vi "Lab Panel V4.82.vi"() -> ()   [LabVIEW 2013] (continued)
                            n2114 = local write "ON L04-2"(w3494) -> ()
                          }
                        }
                      }
                      frame #1 {
                        n2115 = Unbundle(w3502) -> ("amps"=w3501:dbl, "volts"=w3500:dbl, "pf"=w3499:dbl)
                        n2116 = case shown="True" w3503 {
                          tunnel: w3510 -> [_ w3542]
                          tunnel: w3509 -> [_ w3549]
                          tunnel: w3508 -> [_ _]
                          tunnel: w3507 -> [_ _]
                          tunnel: w3506 -> [_ w3548]
                          tunnel: w3505 -> [_ w3547]
                          tunnel: w3504 -> [_ w3512]
                          tunnel: w3501 -> [_ w3544]
                          tunnel: w3500 -> [_ w3543]
                          tunnel: w3499 -> [_ w3541]
                          tunnel: w3498 -> [_ w3533]
                          frame False {
                          }
                          frame True {
                            n2117 = local read "TDMS LAB04-2"() -> (w3546:refnum<k34>)
                            n2118 = Build Array(w3543) -> (w3538:dbl[])
                            n2119 = Build Array(w3541) -> (w3537:dbl[])
                            n2120 = Build Array(w3548) -> (w3536:dbl[])
                            n2121 = Build Array(w3549) -> (w3535:dbl[])
                            n2122 = Build Array(w3544) -> (w3540:dbl[])
                            n2123 = Build Array(w3542) -> (w3539:dbl[])
                            n2124 = Build Array(w3547) -> (w3534:dbl[])
                            n2125 = Build Array("AMPS ON", "AMPS OFF", "VOLTS", "PF", "TEMP Live", "TEMP Neut", "CYCLE") -> (w3517:string[])
                            n2126 = Bundle By Name("Y"=w3540, "t0"=w3533) -> (w3532:waveform(dbl))  [unwired: 1 in]
                            n2127 = Bundle By Name("Y"=w3539, "t0"=w3533) -> (w3531:waveform(dbl))  [unwired: 1 in]
                            n2128 = Bundle By Name("Y"=w3538, "t0"=w3533) -> (w3530:waveform(dbl))  [unwired: 1 in]
                            n2129 = Bundle By Name("Y"=w3537, "t0"=w3533) -> (w3529:waveform(dbl))  [unwired: 1 in]
                            n2130 = Bundle By Name("Y"=w3536, "t0"=w3533) -> (w3528:waveform(dbl))  [unwired: 1 in]
                            n2131 = Bundle By Name("Y"=w3535, "t0"=w3533) -> (w3527:waveform(dbl))  [unwired: 1 in]
                            n2132 = Bundle By Name("Y"=w3534, "t0"=w3533) -> (w3526:waveform(dbl))  [unwired: 1 in]
                            n2133 = Build Array(w3532, w3531, w3530, w3529, w3528, w3527, w3526) -> (w3525:waveform(dbl)[])
                            n2134 = TDMS Write(0:w3546, 5:"TEST VALUES", 7:w3517, 9:w3525) -> (4:w3516:refnum<k34>, 6:w3515:string, 15:w3514:errorcluster)  [unwired: 2 in, 1 out]
                            n2135 = TDMS Write(0:w3516, 5:w3515, 7:"TIME", 9:w3512, 11:w3514) -> (15:w3511:errorcluster)  [unwired: 1 in, 3 out]
                            n2136 = local write "data file error"(w3511) -> ()
                          }
                        }
                      }
                    }
                  }
                }
              }
              frame #8 {
                n2137 = case shown="True" w3550 {
                  tunnel: w3554 -> [_ w3559]
                  tunnel: w3553 -> [_ w3558]
                  tunnel: w3552 -> [_ w3556]
                  tunnel: w3551 -> [_ w3555]
                  frame False {
                  }
                  frame True {
                    n2138 = local read "DISP LAB05-1"() -> (w3560:T4)
                    n2139 = local read "SIG LAB05-1"() -> (w3561:T2)
                    n2140 = local read "ON L05-1"() -> (w3557:cluster{"amps":dbl, "volts":dbl, "pf":dbl})
                    n2141 = Unbundle(w3561) -> ("AMPS"=w3567:dbl, "VOLTS"=w3565:dbl, "PF"=w3564:dbl, "Tmp Live"=w3563:dbl, "Tmp Neut"=w3566:dbl)
                    n2142 = Unbundle(w3560) -> ("CYCLE"=w3562:dbl)  [unwired: 2 out]
                    n2143 = stacked-sequence {
                      tunnel: w3567 -> [w3571 w3590]
                      tunnel: w3566 -> [_ w3589]
                      tunnel: w3565 -> [w3570 w3588]
                      tunnel: w3564 -> [w3569 w3587]
                      tunnel: w3563 -> [_ w3586]
                      tunnel: w3562 -> [_ w3585]
                      tunnel: w3559 -> [_ w3584]
                      tunnel: w3558 -> [w3572 _]
                      tunnel: w3557 -> [w3568 w3582]
                      tunnel: w3556 -> [_ w3583]
                      tunnel: w3555 -> [_ w3578]
                      frame #0 {
                        n2144 = case shown="True" w3572 {
                          tunnel: w3571 -> [_ w3577]
                          tunnel: w3570 -> [_ w3576]
                          tunnel: w3569 -> [_ w3575]
                          tunnel: w3568 -> [_ w3573]
                          frame False {
                          }
                          frame True {
                            n2145 = Bundle(cluster=w3573, "amps"=w3577, "volts"=w3576, "pf"=w3575) -> (w3574:cluster{"amps":dbl, "volts":dbl, "pf":dbl})
                            n2146 = local write "ON L05-1"(w3574) -> ()
                          }
                        }
                      }
                      frame #1 {
                        n2147 = Unbundle(w3582) -> ("amps"=w3581:dbl, "volts"=w3580:dbl, "pf"=w3579:dbl)
                        n2148 = case shown="True" w3583 {
                          tunnel: w3590 -> [_ w3622]
                          tunnel: w3589 -> [_ w3629]
                          tunnel: w3588 -> [_ _]
                          tunnel: w3587 -> [_ _]
                          tunnel: w3586 -> [_ w3628]
                          tunnel: w3585 -> [_ w3627]
                          tunnel: w3584 -> [_ w3592]
                          tunnel: w3581 -> [_ w3624]
                          tunnel: w3580 -> [_ w3623]
                          tunnel: w3579 -> [_ w3621]
                          tunnel: w3578 -> [_ w3613]
                          frame False {
                          }
                          frame True {
                            n2149 = local read "TDMS LAB05-1"() -> (w3626:refnum<k34>)
                            n2150 = Build Array(w3623) -> (w3618:dbl[])
                            n2151 = Build Array(w3621) -> (w3617:dbl[])
                            n2152 = Build Array(w3628) -> (w3616:dbl[])
                            n2153 = Build Array(w3629) -> (w3615:dbl[])
                            n2154 = Build Array(w3624) -> (w3620:dbl[])
                            n2155 = Build Array(w3622) -> (w3619:dbl[])
                            n2156 = Build Array(w3627) -> (w3614:dbl[])
                            n2157 = Build Array("AMPS ON", "AMPS OFF", "VOLTS", "PF", "TEMP Live", "TEMP Neut", "CYCLE") -> (w3597:string[])
                            n2158 = Bundle By Name("Y"=w3620, "t0"=w3613) -> (w3612:waveform(dbl))  [unwired: 1 in]
                            n2159 = Bundle By Name("Y"=w3619, "t0"=w3613) -> (w3611:waveform(dbl))  [unwired: 1 in]
                            n2160 = Bundle By Name("Y"=w3618, "t0"=w3613) -> (w3610:waveform(dbl))  [unwired: 1 in]
                            n2161 = Bundle By Name("Y"=w3617, "t0"=w3613) -> (w3609:waveform(dbl))  [unwired: 1 in]
                            n2162 = Bundle By Name("Y"=w3616, "t0"=w3613) -> (w3608:waveform(dbl))  [unwired: 1 in]
                            n2163 = Bundle By Name("Y"=w3615, "t0"=w3613) -> (w3607:waveform(dbl))  [unwired: 1 in]
                            n2164 = Bundle By Name("Y"=w3614, "t0"=w3613) -> (w3606:waveform(dbl))  [unwired: 1 in]
                            n2165 = Build Array(w3612, w3611, w3610, w3609, w3608, w3607, w3606) -> (w3605:waveform(dbl)[])
                            n2166 = TDMS Write(0:w3626, 5:"TEST VALUES", 7:w3597, 9:w3605) -> (4:w3596:refnum<k34>, 6:w3595:string, 15:w3594:errorcluster)  [unwired: 2 in, 1 out]
                            n2167 = TDMS Write(0:w3596, 5:w3595, 7:"TIME", 9:w3592, 11:w3594) -> (15:w3591:errorcluster)  [unwired: 1 in, 3 out]
                            n2168 = local write "data file error"(w3591) -> ()
                          }
                        }
                      }
                    }
                  }
                }
              }
              frame #9 {
                n2169 = case shown="True" w3630 {
                  tunnel: w3634 -> [_ w3639]
                  tunnel: w3633 -> [_ w3638]
                  tunnel: w3632 -> [_ w3636]
                  tunnel: w3631 -> [_ w3635]
                  frame False {
                  }
                  frame True {
                    n2170 = local read "DISP LAB05-2"() -> (w3640:T4)
                    n2171 = local read "SIG LAB05-2"() -> (w3641:T2)
                    n2172 = local read "ON L05-2"() -> (w3637:cluster{"amps":dbl, "volts":dbl, "pf":dbl})
                    n2173 = Unbundle(w3641) -> ("AMPS"=w3647:dbl, "VOLTS"=w3645:dbl, "PF"=w3644:dbl, "Tmp Live"=w3643:dbl, "Tmp Neut"=w3646:dbl)
                    n2174 = Unbundle(w3640) -> ("CYCLE"=w3642:dbl)  [unwired: 2 out]
                    n2175 = stacked-sequence {
                      tunnel: w3647 -> [w3651 w3670]
                      tunnel: w3646 -> [_ w3669]
                      tunnel: w3645 -> [w3650 w3668]
                      tunnel: w3644 -> [w3649 w3667]
                      tunnel: w3643 -> [_ w3666]
                      tunnel: w3642 -> [_ w3665]
                      tunnel: w3639 -> [_ w3664]
                      tunnel: w3638 -> [w3652 _]
                      tunnel: w3637 -> [w3648 w3662]
                      tunnel: w3636 -> [_ w3663]
                      tunnel: w3635 -> [_ w3658]
                      frame #0 {
                        n2176 = case shown="True" w3652 {
                          tunnel: w3651 -> [_ w3657]
                          tunnel: w3650 -> [_ w3656]
                          tunnel: w3649 -> [_ w3655]
                          tunnel: w3648 -> [_ w3653]
                          frame False {
                          }
                          frame True {
                            n2177 = Bundle(cluster=w3653, "amps"=w3657, "volts"=w3656, "pf"=w3655) -> (w3654:cluster{"amps":dbl, "volts":dbl, "pf":dbl})
                            n2178 = local write "ON L05-2"(w3654) -> ()
                          }
                        }
                      }
                      frame #1 {
                        n2179 = Unbundle(w3662) -> ("amps"=w3661:dbl, "volts"=w3660:dbl, "pf"=w3659:dbl)
                        n2180 = case shown="True" w3663 {
                          tunnel: w3670 -> [_ w3702]
                          tunnel: w3669 -> [_ w3709]
                          tunnel: w3668 -> [_ _]
                          tunnel: w3667 -> [_ _]
                          tunnel: w3666 -> [_ w3708]
                          tunnel: w3665 -> [_ w3707]
                          tunnel: w3664 -> [_ w3672]
                          tunnel: w3661 -> [_ w3704]
                          tunnel: w3660 -> [_ w3703]
                          tunnel: w3659 -> [_ w3701]
                          tunnel: w3658 -> [_ w3693]
                          frame False {
                          }
                          frame True {
                            n2181 = local read "TDMS LAB05-2"() -> (w3706:refnum<k34>)
                            n2182 = Build Array(w3703) -> (w3698:dbl[])
                            n2183 = Build Array(w3701) -> (w3697:dbl[])
                            n2184 = Build Array(w3708) -> (w3696:dbl[])
                            n2185 = Build Array(w3709) -> (w3695:dbl[])
                            n2186 = Build Array(w3704) -> (w3700:dbl[])
                            n2187 = Build Array(w3702) -> (w3699:dbl[])
                            n2188 = Build Array(w3707) -> (w3694:dbl[])
                            n2189 = Build Array("AMPS ON", "AMPS OFF", "VOLTS", "PF", "TEMP Live", "TEMP Neut", "CYCLE") -> (w3677:string[])
                            n2190 = Bundle By Name("Y"=w3700, "t0"=w3693) -> (w3692:waveform(dbl))  [unwired: 1 in]
                            n2191 = Bundle By Name("Y"=w3699, "t0"=w3693) -> (w3691:waveform(dbl))  [unwired: 1 in]
                            n2192 = Bundle By Name("Y"=w3698, "t0"=w3693) -> (w3690:waveform(dbl))  [unwired: 1 in]
                            n2193 = Bundle By Name("Y"=w3697, "t0"=w3693) -> (w3689:waveform(dbl))  [unwired: 1 in]
                            n2194 = Bundle By Name("Y"=w3696, "t0"=w3693) -> (w3688:waveform(dbl))  [unwired: 1 in]
                            n2195 = Bundle By Name("Y"=w3695, "t0"=w3693) -> (w3687:waveform(dbl))  [unwired: 1 in]
                            n2196 = Bundle By Name("Y"=w3694, "t0"=w3693) -> (w3686:waveform(dbl))  [unwired: 1 in]
                            n2197 = Build Array(w3692, w3691, w3690, w3689, w3688, w3687, w3686) -> (w3685:waveform(dbl)[])
                            n2198 = TDMS Write(0:w3706, 5:"TEST VALUES", 7:w3677, 9:w3685) -> (4:w3676:refnum<k34>, 6:w3675:string, 15:w3674:errorcluster)  [unwired: 2 in, 1 out]
                            n2199 = TDMS Write(0:w3676, 5:w3675, 7:"TIME", 9:w3672, 11:w3674) -> (15:w3671:errorcluster)  [unwired: 1 in, 3 out]
                            n2200 = local write "data file error"(w3671) -> ()
                          }
                        }
                      }
                    }
                  }
                }
              }
            }
          }
          frame #13 {
            # "display test values on chart"
            n2201 = case shown="\"OFF CYCLE\"" "Select  Cycle" {
              tunnel: [1 w3715] -> w3710
              frame "ON CYCLE", Default {
              }
              frame "OFF CYCLE" {
                n2202 = local read "on loops"() -> (w3717:dbl)
                n2203 = Add(x=w3717, y=2) -> (x+y=w3715:dbl)
              }
            }
            n2204 = local read "jig cycle"() -> (w3712:dbl)
            n2205 = Equal?(x=w3712, y=w3710) -> (x = y?=w3713:bool)
            n2206 = case shown="True" w3713 {
              frame False {
              }
              frame True {
                n2207 = local read "SIG LAB05-1"() -> (w3759:T2)
                n2208 = local read "SIG LAB04-2"() -> (w3760:T2)
                n2209 = local read "SIG LAB05-2"() -> (w3758:T2)
                n2210 = local read "SIG LAB04-1"() -> (w3761:T2)
                n2211 = local read "SIG LAB03-1"() -> (w3763:T2)
                n2212 = local read "SIG LAB03-2"() -> (w3762:T2)
                n2213 = local read "SIG LAB01-1"() -> (w3767:T2)
                n2214 = local read "SIG LAB02-2"() -> (w3764:T2)
                n2215 = local read "SIG LAB02-1"() -> (w3765:T2)
                n2216 = local read "SIG LAB01-2"() -> (w3766:T2)
                n2217 = Unbundle(w3760) -> ("AMPS"=w3750:dbl, "VOLTS"=w3740:dbl, "Tmp Live"=w3730:dbl, "Tmp Neut"=w3720:dbl)  [unwired: 1 out]
                n2218 = Unbundle(w3759) -> ("AMPS"=w3749:dbl, "VOLTS"=w3739:dbl, "Tmp Live"=w3729:dbl, "Tmp Neut"=w3719:dbl)  [unwired: 1 out]
                n2219 = Unbundle(w3758) -> ("AMPS"=w3748:dbl, "VOLTS"=w3738:dbl, "Tmp Live"=w3728:dbl, "Tmp Neut"=w3718:dbl)  [unwired: 1 out]
                n2220 = Unbundle(w3761) -> ("AMPS"=w3751:dbl, "VOLTS"=w3741:dbl, "Tmp Live"=w3731:dbl, "Tmp Neut"=w3721:dbl)  [unwired: 1 out]
                n2221 = Unbundle(w3762) -> ("AMPS"=w3752:dbl, "VOLTS"=w3742:dbl, "Tmp Live"=w3732:dbl, "Tmp Neut"=w3722:dbl)  [unwired: 1 out]
                n2222 = Unbundle(w3763) -> ("AMPS"=w3753:dbl, "VOLTS"=w3743:dbl, "Tmp Live"=w3733:dbl, "Tmp Neut"=w3723:dbl)  [unwired: 1 out]
                n2223 = Unbundle(w3764) -> ("AMPS"=w3754:dbl, "VOLTS"=w3744:dbl, "Tmp Live"=w3734:dbl, "Tmp Neut"=w3724:dbl)  [unwired: 1 out]
                n2224 = Unbundle(w3765) -> ("AMPS"=w3755:dbl, "VOLTS"=w3745:dbl, "Tmp Live"=w3735:dbl, "Tmp Neut"=w3725:dbl)  [unwired: 1 out]
                n2225 = Unbundle(w3767) -> ("AMPS"=w3757:dbl, "VOLTS"=w3747:dbl, "Tmp Live"=w3737:dbl, "Tmp Neut"=w3727:dbl)  [unwired: 1 out]
                n2226 = Unbundle(w3766) -> ("AMPS"=w3756:dbl, "VOLTS"=w3746:dbl, "Tmp Live"=w3736:dbl, "Tmp Neut"=w3726:dbl)  [unwired: 1 out]
                n2227 = stacked-sequence {
                  tunnel: w3757 -> [w3778 _ _ _]
                  tunnel: w3756 -> [w3777 _ _ _]
                  tunnel: w3755 -> [w3776 _ _ _]
                  tunnel: w3754 -> [w3775 _ _ _]
                  tunnel: w3753 -> [w3774 _ _ _]
                  tunnel: w3752 -> [w3773 _ _ _]
                  tunnel: w3751 -> [w3772 _ _ _]
                  tunnel: w3750 -> [w3771 _ _ _]
                  tunnel: w3749 -> [w3770 _ _ _]
                  tunnel: w3748 -> [w3769 _ _ _]
                  tunnel: w3747 -> [_ w3789 _ _]
                  tunnel: w3746 -> [_ w3788 _ _]
                  tunnel: w3745 -> [_ w3787 _ _]
                  tunnel: w3744 -> [_ w3786 _ _]
                  tunnel: w3743 -> [_ w3785 _ _]
                  tunnel: w3742 -> [_ w3784 _ _]
                  tunnel: w3741 -> [_ w3783 _ _]
                  tunnel: w3740 -> [_ w3782 _ _]
                  tunnel: w3739 -> [_ w3781 _ _]
                  tunnel: w3738 -> [_ w3780 _ _]
                  tunnel: w3737 -> [_ _ w3800 _]
                  tunnel: w3736 -> [_ _ w3799 _]
                  tunnel: w3735 -> [_ _ w3798 _]
                  tunnel: w3734 -> [_ _ w3797 _]
                  tunnel: w3733 -> [_ _ w3796 _]
                  tunnel: w3732 -> [_ _ w3795 _]
                  tunnel: w3731 -> [_ _ w3794 _]
                  tunnel: w3730 -> [_ _ w3793 _]
                  tunnel: w3729 -> [_ _ w3792 _]
                  tunnel: w3728 -> [_ _ w3791 _]
                  tunnel: w3727 -> [_ _ _ w3811]
                  tunnel: w3726 -> [_ _ _ w3810]
                  tunnel: w3725 -> [_ _ _ w3809]
                  tunnel: w3724 -> [_ _ _ w3808]
                  tunnel: w3723 -> [_ _ _ w3807]
                  tunnel: w3722 -> [_ _ _ w3806]
                  tunnel: w3721 -> [_ _ _ w3805]
                  tunnel: w3720 -> [_ _ _ w3804]
                  tunnel: w3719 -> [_ _ _ w3803]
                  tunnel: w3718 -> [_ _ _ w3802]
                  frame #0 {
                    n2228 = Bundle("AMPS"=w3778, "AMPS"=w3777, "AMPS"=w3776, "AMPS"=w3775, "AMPS"=w3774, "AMPS"=w3773, "AMPS"=w3772, "AMPS"=w3771, "AMPS"=w3770, "AMPS"=w3769) -> (→"TEST AMPS CHART":T6)  [unwired: 1 in]
                  }
                  frame #1 {
                    n2229 = Bundle("VOLTS"=w3789, "VOLTS"=w3788, "VOLTS"=w3787, "VOLTS"=w3786, "VOLTS"=w3785, "VOLTS"=w3784, "VOLTS"=w3783, "VOLTS"=w3782, "VOLTS"=w3781, "VOLTS"=w3780) -> (→"TEST VOLTS CHART":T29)  [unwired: 1 in]
                  }
                  frame #2 {
                    n2230 = Bundle("Tmp Live"=w3800, "Tmp Live"=w3799, "Tmp Live"=w3798, "Tmp Live"=w3797, "Tmp Live"=w3796, "Tmp Live"=w3795, "Tmp Live"=w3794, "Tmp Live"=w3793, "Tmp Live"=w3792, "Tmp Live"=w3791) -> (→"TEMPERATURE (L) CHART":T30)  [unwired: 1 in]
                  }
                  frame #3 {
                    n2231 = Bundle("Tmp Neut"=w3811, "Tmp Neut"=w3810, "Tmp Neut"=w3809, "Tmp Neut"=w3808, "Tmp Neut"=w3807, "Tmp Neut"=w3806, "Tmp Neut"=w3805, "Tmp Neut"=w3804, "Tmp Neut"=w3803, "Tmp Neut"=w3802) -> (→"TEMPERATURE (N) CHART":T31)  [unwired: 1 in]
                  }
                }
              }
            }
          }
          frame #14 {
            # "check for amps fail"
            # "check for cycle test & temperature rise fail conditions"
            n2232 = local read "on loops"() -> (w3838:dbl)
            n2233 = local read "jig cycle"() -> (w3835:dbl)
            n2234 = local read "jig cycle"() -> (w3840:dbl)
            n2235 = Add(x=w3838, y=3.0) -> (x+y=w3836:dbl)
            n2236 = Equal?(x=w3835, y=w3836) -> (x = y?=w3831:bool)
            n2237 = local read "Fail Loops"() -> (w3812:dbl)
            n2238 = Equal?(x=w3840, y=1.0) -> (x = y?=w3833:bool)
            n2239 = global write "Global 1.vi" "fail count"(w3812) -> ()
            n2240 = stacked-sequence {
              tunnel: w3834 -> [w3843 _ _ _ _ _ _ _ _ _]
              tunnel: w3833 -> [w3844 w3864 w3884 w3904 w3924 w3944 w3964 w3984 w4004 w4024]
              tunnel: w3832 -> [w3841 _ _ _ _ _ _ _ _ _]
              tunnel: w3831 -> [w3842 w3863 w3883 w3903 w3923 w3943 w3963 w3983 w4003 w4023]
              tunnel: w3830 -> [_ w3862 _ _ _ _ _ _ _ _]
              tunnel: w3829 -> [_ w3861 _ _ _ _ _ _ _ _]
              tunnel: w3828 -> [_ _ w3882 _ _ _ _ _ _ _]
              tunnel: w3827 -> [_ _ w3881 _ _ _ _ _ _ _]
              tunnel: w3826 -> [_ _ _ w3902 _ _ _ _ _ _]
              tunnel: w3825 -> [_ _ _ w3901 _ _ _ _ _ _]
              tunnel: w3824 -> [_ _ _ _ w3922 _ _ _ _ _]
              tunnel: w3823 -> [_ _ _ _ w3921 _ _ _ _ _]
              tunnel: w3822 -> [_ _ _ _ _ w3942 _ _ _ _]
              tunnel: w3821 -> [_ _ _ _ _ w3941 _ _ _ _]
              tunnel: w3820 -> [_ _ _ _ _ _ w3962 _ _ _]
              tunnel: w3819 -> [_ _ _ _ _ _ w3961 _ _ _]
              tunnel: w3818 -> [_ _ _ _ _ _ _ w3982 _ _]
              tunnel: w3817 -> [_ _ _ _ _ _ _ w3981 _ _]
              tunnel: w3816 -> [_ _ _ _ _ _ _ _ w4002 _]
              tunnel: w3815 -> [_ _ _ _ _ _ _ _ w4001 _]
              tunnel: w3814 -> [_ _ _ _ _ _ _ _ _ w4022]
              tunnel: w3813 -> [_ _ _ _ _ _ _ _ _ w4021]
              frame #0 {
                # "LAB01-1"
                n2241 = case shown="True" w3841 {
                  tunnel: w3844 -> [_ w3857]
                  tunnel: w3843 -> [_ w3854]
                  tunnel: w3842 -> [_ w3853]
                  frame False {
                  }
                  frame True {
                    n2242 = local read "TEMP START LAB01-1"() -> (w3859:cluster{"TL":dbl, "TN":dbl})
                    n2243 = local read "RESULT LAB01-1"() -> (w3848:bool)
                    n2244 = local read "FAIL LAB01-1"() -> (w3851:cluster{"LO":dbl, "HI":dbl})
                    n2245 = local read "TDMS LAB01-1"() -> (w3858:refnum<k34>)
                    n2246 = local read "SET LAB01-1"() -> (w3855:T5)
                    n2247 = local read "DISP LAB01-1"() -> (w3856:T4)
                    n2248 = local read "SIG LAB01-1"() -> (w3860:T2)
                    n2249 = Bundle("FAIL LAB01-1"=w3851, "SIG LAB01-1"=w3860, "TEMP START LAB01-1"=w3859, "DISP LAB01-1"=w3856, "SET LAB01-1"=w3855, "TDMS LAB01-1"=w3858) -> (w3845:T32)  [unwired: 1 in]
                    n2250 = call "sub vi - cycle&temp fail v6.vi"("Amps Lo?"=w3857, "Input Cluster"=w3845, "SELECT"=w3854, "Amps Hi?"=w3853, "Result In"=w3848) -> ("(FAIL) out"=w3850:cluster{"FAIL LO":dbl, "FAIL HI":dbl}, "(DISP) out"=w3846:T4, "T-RISE"=w3847:cluster{"T-RISE (L)":dbl, "T-RISE (N)":dbl}, "Result Out"=w3849:bool, "file error"=w3852:errorcluster)  [unwired: 10 in]
                    n2251 = local write "TEMP RISE LAB01-1"(w3847) -> ()
                    n2252 = local write "FAIL LAB01-1"(w3850) -> ()
                    n2253 = local write "DISP LAB01-1"(w3846) -> ()
                    n2254 = local write "RESULT LAB01-1"(w3849) -> ()
                    n2255 = local write "data file error"(w3852) -> ()
                  }
                }
              }
              frame #1 {
                # "LAB01-2"
                n2256 = case shown="True" w3862 {
                  tunnel: w3864 -> [_ w3877]
                  tunnel: w3861 -> [_ w3874]
                  tunnel: w3863 -> [_ w3873]
                  frame False {
                  }
                  frame True {
                    n2257 = local read "TEMP START LAB01-2"() -> (w3879:cluster{"TL":dbl, "TN":dbl})
                    n2258 = local read "FAIL LAB01-2"() -> (w3870:cluster{"LO":dbl, "HI":dbl})
                    n2259 = local read "TDMS LAB01-2"() -> (w3878:refnum<k34>)
                    n2260 = local read "SET LAB01-2"() -> (w3875:T5)
                    n2261 = local read "DISP LAB01-2"() -> (w3876:T4)
                    n2262 = local read "RESULT LAB01-2"() -> (w3867:bool)
                    n2263 = local read "SIG LAB01-2"() -> (w3880:T2)
                    n2264 = Bundle("FAIL LAB01-2"=w3870, "SIG LAB01-2"=w3880, "TEMP START LAB01-2"=w3879, "DISP LAB01-2"=w3876, "SET LAB01-2"=w3875, "TDMS LAB01-2"=w3878) -> (w3865:T33)  [unwired: 1 in]
                    n2265 = call "sub vi - cycle&temp fail v6.vi"("Amps Lo?"=w3877, "Input Cluster"=w3865, "SELECT"=w3874, "Amps Hi?"=w3873, "Result In"=w3867) -> ("(FAIL) out"=w3869:cluster{"FAIL LO":dbl, "FAIL HI":dbl}, "(DISP) out"=w3872:T4, "T-RISE"=w3866:cluster{"T-RISE (L)":dbl, "T-RISE (N)":dbl}, "Result Out"=w3868:bool, "file error"=w3871:errorcluster)  [unwired: 10 in]
                    n2266 = local write "TEMP RISE LAB01-2"(w3866) -> ()
                    n2267 = local write "FAIL LAB01-2"(w3869) -> ()
                    n2268 = local write "DISP LAB01-2"(w3872) -> ()
                    n2269 = local write "RESULT LAB01-2"(w3868) -> ()
                    n2270 = local write "data file error"(w3871) -> ()
                  }
                }
              }
              frame #2 {
                # "LAB02-1"
                n2271 = case shown="True" w3882 {
                  tunnel: w3884 -> [_ w3897]
                  tunnel: w3881 -> [_ w3894]
                  tunnel: w3883 -> [_ w3893]
                  frame False {
                  }
                  frame True {
                    n2272 = local read "TEMP START LAB02-1"() -> (w3899:cluster{"TL":dbl, "TN":dbl})
                    n2273 = local read "FAIL LAB02-1"() -> (w3890:cluster{"LO":dbl, "HI":dbl})
                    n2274 = local read "TDMS LAB02-1"() -> (w3898:refnum<k34>)
                    n2275 = local read "SET LAB02-1"() -> (w3895:T5)
                    n2276 = local read "DISP LAB02-1"() -> (w3896:T4)
                    n2277 = local read "SIG LAB02-1"() -> (w3900:T2)
                    n2278 = local read "RESULT LAB02-1"() -> (w3887:bool)
                    n2279 = Bundle("FAIL LAB02-1"=w3890, "SIG LAB02-1"=w3900, "TEMP START LAB02-1"=w3899, "DISP LAB02-1"=w3896, "SET LAB02-1"=w3895, "TDMS LAB02-1"=w3898) -> (w3885:T34)  [unwired: 1 in]
                    n2280 = call "sub vi - cycle&temp fail v6.vi"("Amps Lo?"=w3897, "Input Cluster"=w3885, "SELECT"=w3894, "Amps Hi?"=w3893, "Result In"=w3887) -> ("(FAIL) out"=w3889:cluster{"FAIL LO":dbl, "FAIL HI":dbl}, "(DISP) out"=w3892:T4, "T-RISE"=w3886:cluster{"T-RISE (L)":dbl, "T-RISE (N)":dbl}, "Result Out"=w3888:bool, "file error"=w3891:errorcluster)  [unwired: 10 in]
                    n2281 = local write "TEMP RISE LAB02-1"(w3886) -> ()
                    n2282 = local write "FAIL LAB02-1"(w3889) -> ()
                    n2283 = local write "DISP LAB02-1"(w3892) -> ()
                    n2284 = local write "RESULT LAB02-1"(w3888) -> ()
                    n2285 = local write "data file error"(w3891) -> ()
                  }
                }
              }
              frame #3 {
                # "LAB02-2"
                n2286 = case shown="True" w3902 {
                  tunnel: w3904 -> [_ w3917]
                  tunnel: w3901 -> [_ w3914]
                  tunnel: w3903 -> [_ w3913]
                  frame False {
                  }
                  frame True {
                    n2287 = local read "TEMP START LAB02-2"() -> (w3919:cluster{"TL":dbl, "TN":dbl})
                    n2288 = local read "FAIL LAB02-2"() -> (w3910:cluster{"LO":dbl, "HI":dbl})
                    n2289 = local read "TDMS LAB02-2"() -> (w3918:refnum<k34>)
                    n2290 = local read "SET LAB02-2"() -> (w3915:T5)
                    n2291 = local read "DISP LAB02-2"() -> (w3916:T4)
                    n2292 = local read "SIG LAB02-2"() -> (w3920:T2)
                    n2293 = local read "RESULT LAB02-2"() -> (w3907:bool)
                    n2294 = Bundle("FAIL LAB02-2"=w3910, "SIG LAB02-2"=w3920, "TEMP START LAB02-2"=w3919, "DISP LAB02-2"=w3916, "SET LAB02-2"=w3915, "TDMS LAB02-2"=w3918) -> (w3905:T35)  [unwired: 1 in]
                    n2295 = call "sub vi - cycle&temp fail v6.vi"("Amps Lo?"=w3917, "Input Cluster"=w3905, "SELECT"=w3914, "Amps Hi?"=w3913, "Result In"=w3907) -> ("(FAIL) out"=w3909:cluster{"FAIL LO":dbl, "FAIL HI":dbl}, "(DISP) out"=w3912:T4, "T-RISE"=w3906:cluster{"T-RISE (L)":dbl, "T-RISE (N)":dbl}, "Result Out"=w3908:bool, "file error"=w3911:errorcluster)  [unwired: 10 in]
                    n2296 = local write "TEMP RISE LAB02-2"(w3906) -> ()
                    n2297 = local write "FAIL LAB02-2"(w3909) -> ()
                    n2298 = local write "DISP LAB02-2"(w3912) -> ()
                    n2299 = local write "RESULT LAB02-2"(w3908) -> ()
                    n2300 = local write "data file error"(w3911) -> ()
                  }
                }
              }
              frame #4 {
                # "LAB03-1"
                n2301 = case shown="True" w3922 {
                  tunnel: w3924 -> [_ w3937]
                  tunnel: w3921 -> [_ w3934]
                  tunnel: w3923 -> [_ w3933]
                  frame False {
                  }
                  frame True {
                    n2302 = local read "TEMP START LAB03-1"() -> (w3939:cluster{"TL":dbl, "TN":dbl})
                    n2303 = local read "FAIL LAB03-1"() -> (w3930:cluster{"LO":dbl, "HI":dbl})
                    n2304 = local read "TDMS LAB03-1"() -> (w3938:refnum<k34>)
                    n2305 = local read "SET LAB03-1"() -> (w3935:T5)
                    n2306 = local read "DISP LAB03-1"() -> (w3936:T4)
                    n2307 = local read "SIG LAB03-1"() -> (w3940:T2)
                    n2308 = local read "RESULT LAB03-1"() -> (w3927:bool)
                    n2309 = Bundle("FAIL LAB03-1"=w3930, "SIG LAB03-1"=w3940, "TEMP START LAB03-1"=w3939, "DISP LAB03-1"=w3936, "SET LAB03-1"=w3935, "TDMS LAB03-1"=w3938) -> (w3925:T36)  [unwired: 1 in]
                    n2310 = call "sub vi - cycle&temp fail v6.vi"("Amps Lo?"=w3937, "Input Cluster"=w3925, "SELECT"=w3934, "Amps Hi?"=w3933, "Result In"=w3927) -> ("(FAIL) out"=w3929:cluster{"FAIL LO":dbl, "FAIL HI":dbl}, "(DISP) out"=w3932:T4, "T-RISE"=w3926:cluster{"T-RISE (L)":dbl, "T-RISE (N)":dbl}, "Result Out"=w3928:bool, "file error"=w3931:errorcluster)  [unwired: 10 in]
                    n2311 = local write "TEMP RISE LAB03-1"(w3926) -> ()
                    n2312 = local write "FAIL LAB03-1"(w3929) -> ()
                    n2313 = local write "DISP LAB03-1"(w3932) -> ()
                    n2314 = local write "RESULT LAB03-1"(w3928) -> ()
                    n2315 = local write "data file error"(w3931) -> ()
                  }
                }
              }
              frame #5 {
                # "LAB03-2"
                n2316 = case shown="True" w3942 {
                  tunnel: w3944 -> [_ w3957]
                  tunnel: w3941 -> [_ w3954]
                  tunnel: w3943 -> [_ w3953]
                  frame False {
                  }
                  frame True {
                    n2317 = local read "TEMP START LAB03-2"() -> (w3959:cluster{"TL":dbl, "TN":dbl})
                    n2318 = local read "FAIL LAB03-2"() -> (w3950:cluster{"LO":dbl, "HI":dbl})
                    n2319 = local read "TDMS LAB03-2"() -> (w3958:refnum<k34>)
                    n2320 = local read "SET LAB03-2"() -> (w3955:T5)
                    n2321 = local read "DISP LAB03-2"() -> (w3956:T4)
                    n2322 = local read "RESULT LAB03-2"() -> (w3947:bool)
                    n2323 = local read "SIG LAB03-2"() -> (w3960:T2)
                    n2324 = Bundle("FAIL LAB03-2"=w3950, "SIG LAB03-2"=w3960, "TEMP START LAB03-2"=w3959, "DISP LAB03-2"=w3956, "SET LAB03-2"=w3955, "TDMS LAB03-2"=w3958) -> (w3945:T37)  [unwired: 1 in]
                    n2325 = call "sub vi - cycle&temp fail v6.vi"("Amps Lo?"=w3957, "Input Cluster"=w3945, "SELECT"=w3954, "Amps Hi?"=w3953, "Result In"=w3947) -> ("(FAIL) out"=w3949:cluster{"FAIL LO":dbl, "FAIL HI":dbl}, "(DISP) out"=w3952:T4, "T-RISE"=w3946:cluster{"T-RISE (L)":dbl, "T-RISE (N)":dbl}, "Result Out"=w3948:bool, "file error"=w3951:errorcluster)  [unwired: 10 in]
                    n2326 = local write "FAIL LAB03-2"(w3949) -> ()
                    n2327 = local write "TEMP RISE LAB03-2"(w3946) -> ()
                    n2328 = local write "DISP LAB03-2"(w3952) -> ()
                    n2329 = local write "RESULT LAB03-2"(w3948) -> ()
                    n2330 = local write "data file error"(w3951) -> ()
                  }
                }
              }
              frame #6 {
                # "LAB04-1"
                n2331 = case shown="True" w3962 {
                  tunnel: w3964 -> [_ w3977]
                  tunnel: w3961 -> [_ w3974]
                  tunnel: w3963 -> [_ w3973]
                  frame False {
                  }
                  frame True {
                    n2332 = local read "TEMP START LAB04-1"() -> (w3979:cluster{"TL":dbl, "TN":dbl})
                    n2333 = local read "FAIL LAB04-1"() -> (w3970:cluster{"LO":dbl, "HI":dbl})
                    n2334 = local read "TDMS LAB04-1"() -> (w3978:refnum<k34>)
                    n2335 = local read "SET LAB04-1"() -> (w3975:T5)
                    n2336 = local read "DISP LAB04-1"() -> (w3976:T4)
                    n2337 = local read "SIG LAB04-1"() -> (w3980:T2)
                    n2338 = local read "RESULT LAB04-1"() -> (w3967:bool)
                    n2339 = Bundle("FAIL LAB04-1"=w3970, "SIG LAB04-1"=w3980, "TEMP START LAB04-1"=w3979, "DISP LAB04-1"=w3976, "SET LAB04-1"=w3975, "TDMS LAB04-1"=w3978) -> (w3965:T38)  [unwired: 1 in]
                    n2340 = call "sub vi - cycle&temp fail v6.vi"("Amps Lo?"=w3977, "Input Cluster"=w3965, "SELECT"=w3974, "Amps Hi?"=w3973, "Result In"=w3967) -> ("(FAIL) out"=w3969:cluster{"FAIL LO":dbl, "FAIL HI":dbl}, "(DISP) out"=w3972:T4, "T-RISE"=w3966:cluster{"T-RISE (L)":dbl, "T-RISE (N)":dbl}, "Result Out"=w3968:bool, "file error"=w3971:errorcluster)  [unwired: 10 in]
                    n2341 = local write "TEMP RISE LAB04-1"(w3966) -> ()
                    n2342 = local write "FAIL LAB04-1"(w3969) -> ()
                    n2343 = local write "DISP LAB04-1"(w3972) -> ()
                    n2344 = local write "RESULT LAB04-1"(w3968) -> ()
                    n2345 = local write "data file error"(w3971) -> ()
                  }
                }
              }
              frame #7 {
                # "LAB04-2"
                n2346 = case shown="True" w3982 {
                  tunnel: w3984 -> [_ w3997]
                  tunnel: w3981 -> [_ w3994]
                  tunnel: w3983 -> [_ w3993]
                  frame False {
                  }
                  frame True {
                    n2347 = local read "TEMP START LAB04-2"() -> (w3999:cluster{"TL":dbl, "TN":dbl})
                    n2348 = local read "FAIL LAB04-2"() -> (w3990:cluster{"LO":dbl, "HI":dbl})
                    n2349 = local read "TDMS LAB04-2"() -> (w3998:refnum<k34>)
                    n2350 = local read "SET LAB04-2"() -> (w3995:T5)
                    n2351 = local read "DISP LAB04-2"() -> (w3996:T4)
                    n2352 = local read "SIG LAB04-2"() -> (w4000:T2)
                    n2353 = local read "RESULT LAB04-2"() -> (w3987:bool)
                    n2354 = Bundle("FAIL LAB04-2"=w3990, "SIG LAB04-2"=w4000, "TEMP START LAB04-2"=w3999, "DISP LAB04-2"=w3996, "SET LAB04-2"=w3995, "TDMS LAB04-2"=w3998) -> (w3985:T39)  [unwired: 1 in]
                    n2355 = call "sub vi - cycle&temp fail v6.vi"("Amps Lo?"=w3997, "Input Cluster"=w3985, "SELECT"=w3994, "Amps Hi?"=w3993, "Result In"=w3987) -> ("(FAIL) out"=w3989:cluster{"FAIL LO":dbl, "FAIL HI":dbl}, "(DISP) out"=w3992:T4, "T-RISE"=w3986:cluster{"T-RISE (L)":dbl, "T-RISE (N)":dbl}, "Result Out"=w3988:bool, "file error"=w3991:errorcluster)  [unwired: 10 in]
                    n2356 = local write "TEMP RISE LAB04-2"(w3986) -> ()
                    n2357 = local write "FAIL LAB04-2"(w3989) -> ()
                    n2358 = local write "DISP LAB04-2"(w3992) -> ()
                    n2359 = local write "RESULT LAB04-2"(w3988) -> ()
                    n2360 = local write "data file error"(w3991) -> ()
                  }
                }
              }
              frame #8 {
                # "LAB05-1"
                n2361 = case shown="True" w4002 {
                  tunnel: w4004 -> [_ w4017]
                  tunnel: w4001 -> [_ w4014]
                  tunnel: w4003 -> [_ w4013]
                  frame False {
                  }
                  frame True {
                    n2362 = local read "TEMP START LAB05-1"() -> (w4019:cluster{"TL":dbl, "TN":dbl})
                    n2363 = local read "FAIL LAB05-1"() -> (w4010:cluster{"LO":dbl, "HI":dbl})
                    n2364 = local read "TDMS LAB05-1"() -> (w4018:refnum<k34>)
                    n2365 = local read "SET LAB05-1"() -> (w4015:T5)
                    n2366 = local read "DISP LAB05-1"() -> (w4016:T4)
                    n2367 = local read "SIG LAB05-1"() -> (w4020:T2)
                    n2368 = local read "RESULT LAB05-1"() -> (w4007:bool)
                    n2369 = Bundle("FAIL LAB05-1"=w4010, "SIG LAB05-1"=w4020, "TEMP START LAB05-1"=w4019, "DISP LAB05-1"=w4016, "SET LAB05-1"=w4015, "TDMS LAB05-1"=w4018) -> (w4005:T40)  [unwired: 1 in]
                    n2370 = call "sub vi - cycle&temp fail v6.vi"("Amps Lo?"=w4017, "Input Cluster"=w4005, "SELECT"=w4014, "Amps Hi?"=w4013, "Result In"=w4007) -> ("(FAIL) out"=w4009:cluster{"FAIL LO":dbl, "FAIL HI":dbl}, "(DISP) out"=w4012:T4, "T-RISE"=w4006:cluster{"T-RISE (L)":dbl, "T-RISE (N)":dbl}, "Result Out"=w4008:bool, "file error"=w4011:errorcluster)  [unwired: 10 in]
                    n2371 = local write "TEMP RISE LAB05-1"(w4006) -> ()
                    n2372 = local write "FAIL LAB05-1"(w4009) -> ()
                    n2373 = local write "DISP LAB05-1"(w4012) -> ()
                    n2374 = local write "RESULT LAB05-1"(w4008) -> ()
                    n2375 = local write "data file error"(w4011) -> ()
                  }
                }
              }
              frame #9 {
                # "LAB05-2"
                n2376 = case shown="True" w4022 {
                  tunnel: w4024 -> [_ w4037]
                  tunnel: w4021 -> [_ w4034]
                  tunnel: w4023 -> [_ w4033]
                  frame False {
                  }
                  frame True {
                    n2377 = local read "TEMP START LAB05-2"() -> (w4039:cluster{"TL":dbl, "TN":dbl})
                    n2378 = local read "FAIL LAB05-2"() -> (w4030:cluster{"LO":dbl, "HI":dbl})
                    n2379 = local read "TDMS LAB05-2"() -> (w4038:refnum<k34>)
                    n2380 = local read "SET LAB05-2"() -> (w4035:T5)
                    n2381 = local read "DISP LAB05-2"() -> (w4036:T4)
                    n2382 = local read "SIG LAB05-2"() -> (w4040:T2)
                    n2383 = local read "RESULT LAB05-2"() -> (w4027:bool)
                    n2384 = Bundle("FAIL LAB05-2"=w4030, "SIG LAB05-2"=w4040, "TEMP START LAB05-2"=w4039, "DISP LAB05-2"=w4036, "SET LAB05-2"=w4035, "TDMS LAB05-2"=w4038) -> (w4025:T41)  [unwired: 1 in]
                    n2385 = call "sub vi - cycle&temp fail v6.vi"("Amps Lo?"=w4037, "Input Cluster"=w4025, "SELECT"=w4034, "Amps Hi?"=w4033, "Result In"=w4027) -> ("(FAIL) out"=w4029:cluster{"FAIL LO":dbl, "FAIL HI":dbl}, "(DISP) out"=w4032:T4, "T-RISE"=w4026:cluster{"T-RISE (L)":dbl, "T-RISE (N)":dbl}, "Result Out"=w4028:bool, "file error"=w4031:errorcluster)  [unwired: 10 in]
                    n2386 = local write "TEMP RISE LAB05-2"(w4026) -> ()
                    n2387 = local write "FAIL LAB05-2"(w4029) -> ()
                    n2388 = local write "DISP LAB05-2"(w4032) -> ()
                    n2389 = local write "RESULT LAB05-2"(w4028) -> ()
                    n2390 = local write "data file error"(w4031) -> ()
                  }
                }
              }
            }
          }
          frame #15 {
            # "run calibration routine"
            n2391 = local read "CALIBRATE"() -> (w4041:bool)
            n2392 = case shown="True" w4041 {
              frame False {
              }
              frame True {
                n2393 = stacked-sequence {
                  seq-local: [w4042 _ _] -> [_ w4044 _]
                  frame #0 {
                    n2394 = call "CALIBRATION PASSWORD"() -> ("PASSWORD"=w4042:string)  [unwired: 17 in, 2 out]
                  }
                  frame #1 {
                    n2395 = Equal?(x=w4044, y="7777") -> (x = y?=w4043:bool)
                    n2396 = case shown="True" w4043 {
                      frame False {
                      }
                      frame True {
                        n2397 = stacked-sequence {
                          frame #0 {
                            n2398 = call "sub vi - calibration v1.vi"() -> ()  [unwired: 12 in]
                          }
                          frame #1 {
                            n2399 = call "sub vi - get calibration values v1.vi"() -> ("LAB01 (CAL)"=w4050:T8, "LAB02 (CAL)"=w4049:T9, "LAB03 (CAL)"=w4048:T8, "LAB04 (CAL)"=w4047:T8, "calibration file error out"=w4051:errorcluster, "LAB05 (CAL)"=w4046:T8)  [unwired: 10 in]
                            n2400 = local write "calibration file error out"(w4051) -> ()
                            n2401 = local write "CAL LAB04"(w4047) -> ()
                            n2402 = local write "CAL LAB05"(w4046) -> ()
                            n2403 = local write "CAL LAB01"(w4050) -> ()
                            n2404 = local write "CAL LAB02"(w4049) -> ()
                            n2405 = local write "CAL LAB03"(w4048) -> ()
                          }
                        }
                      }
                    }
                  }
                  frame #2 {
                    n2406 = local write "CALIBRATE"(FALSE) -> ()
                  }
                }
              }
            }
          }
          frame #16 {
            # "save certain settings to file"
            n2407 = String To Path(string="c:\\crabtree\\Set Up\\") -> (path=w4054:path)
            n2408 = Build Path(base path=w4054, name or relative path="settings.bin") -> (appended path=w4056:path)
            n2409 = Build Path(base path=w4054, name or relative path="mail.bin") -> (appended path=w4053:path)
            n2410 = Create Folder(path (use dialog)=w4054) -> (error out=w4059:errorcluster)  [unwired: 2 in, 2 out]
            n2411 = call <vilib>:"Clear Errors.vi"("error in (no error)"=w4059) -> ()  [unwired: 6 in, 1 out]
            n2412 = stacked-sequence {
              seq-local: [w4069 _] -> [_ w4082]
              tunnel: w4056 -> [_ w4083]
              tunnel: w4053 -> [_ w4081]
              frame #0 {
                n2413 = local read "C drive data root dir"() -> (w4068:path)
                n2414 = local read "Select COM port"() -> (w4065:refnum<visa-resource-name>)
                n2415 = local read "Network Directory"() -> (w4074:path)
                n2416 = local read "SET LAB05-2"() -> (w4073:T5)
                n2417 = local read "SET LAB05-1"() -> (w4072:T5)
                n2418 = local read "SET LAB04-2"() -> (w4071:T5)
                n2419 = local read "SET LAB03-2"() -> (w4075:T5)
                n2420 = local read "SET LAB04-1"() -> (w4070:T5)
                n2421 = local read "SET LAB03-1"() -> (w4076:T5)
                n2422 = local read "SET LAB02-2"() -> (w4077:T5)
                n2423 = local read "SET LAB02-1"() -> (w4078:T5)
                n2424 = local read "Temp Delay Lps"() -> (w4064:dbl)
                n2425 = local read "SET LAB01-2"() -> (w4079:T5)
                n2426 = local read "Temp Test Cal"() -> (w4061:dbl)
                n2427 = local read "SET LAB01-1"() -> (w4080:T5)
                n2428 = local read "Set Temp Lps"() -> (w4060:dbl)
                n2429 = local read "Temp Value"() -> (w4063:dbl)
                n2430 = local read "Fail Loops"() -> (w4062:dbl)
                n2431 = local read "RATE (Hz)"() -> (w4067:dbl)
                n2432 = local read "SAMPLES"() -> (w4066:dbl)
                n2433 = Bundle("SET LAB01-1"=w4080, "SET LAB01-2"=w4079, "SET LAB02-1"=w4078, "SET LAB02-2"=w4077, "SET LAB03-1"=w4076, "SET LAB03-2"=w4075, "SET LAB04-1"=w4070, "SET LAB04-2"=w4071, "SET LAB05-1"=w4072, "SET LAB05-2"=w4073, "Network Directory"=w4074, "C drive data root dir"=w4068, "RATE (Hz)"=w4067, "SAMPLES"=w4066, "Select COM port"=w4065, "Temp Delay Lps"=w4064, "Temp Value"=w4063, "Fail Loops"=w4062, "Temp Test Cal"=w4061, "Set Temp Lps"=w4060) -> (w4069:T21)  [unwired: 1 in]
              }
              frame #1 {
                n2434 = event shown="[1] \"SET LAB01-1\", \"SET LAB01-2\", \"SET LAB02-1\", \"SET LAB02-2\", \"SET LAB03-1\", \"SET LAB03-2\", \"SET LAB04-1\", \"SET LAB04-2\", \"SET LAB05-1\", \"SET LAB05-2\", \"Network Directory\", \"C drive data root dir\", \"RATE (Hz)\", \"SAMPLES\", \"Select COM port\", \"Temp Delay Lps\", \"Temp Value\", \"Fail Loops\", \"Temp Test Cal\", \"Set Temp Lps\": Value Change" {
                  selector: _ -> [_ _ _]
                  dyn-events: _ -> [_ _ _]
                  timeout: 10.0 -> [_ _ _]
                  tunnel: w4083 -> [_ w4085 _]
                  tunnel: w4082 -> [_ w4086 _]
                  tunnel: w4081 -> [_ _ w4097]
                  event Timeout {
                    n2435 = event-data() -> ()  [unwired: 1 in, 3 out]
                  }
                  event "SET LAB01-1", "SET LAB01-2", "SET LAB02-1", "SET LAB02-2", "SET LAB03-1", "SET LAB03-2", "SET LAB04-1", "SET LAB04-2", "SET LAB05-1", "SET LAB05-2", "Network Directory", "C drive data root dir", "RATE (Hz)", "SAMPLES", "Select COM port", "Temp Delay Lps", "Temp Value", "Fail Loops", "Temp Test Cal", "Set Temp Lps": Value Change {
                    n2436 = event-data() -> ()  [unwired: 1 in, 6 out]
                    n2437 = Open/Create/Replace File(file path (use dialog)=w4085, operation (0:open)=T20."replace or create") -> (refnum out=w4091:refnum<file>, error out=w4090:errorcluster)  [unwired: 4 in, 1 out]
                    n2438 = Write to Binary File(file (use dialog)=w4091, data=w4086, error in=w4090) -> (refnum out=w4089:refnum<file>, error out=w4088:errorcluster)  [unwired: 3 in, 1 out]
                    n2439 = Close File(refnum=w4089, error in=w4088) -> (error out=w4087:errorcluster)  [unwired: 1 out]
                    n2440 = local write "data file error"(w4087) -> ()
                  }
                  event "MAIL SETTINGS.OUT SERVER ADDRESS", "MAIL SETTINGS.FROM ACCOUNT", "MAIL SETTINGS.USER NAME", "MAIL SETTINGS.PASSWORD", "Auto Mail Send", "TO (string):": Value Change {
                    n2441 = event-data() -> ()  [unwired: 1 in, 6 out]
                    n2442 = local read "MAIL SETTINGS"() -> (w4096:T7)
                    n2443 = local read "Auto Mail Send"() -> (w4094:bool)
                    n2444 = local read "TO (string):"() -> (w4093:string)
                    n2445 = Open/Create/Replace File(file path (use dialog)=w4097, operation (0:open)=T20."replace or create") -> (refnum out=w4102:refnum<file>, error out=w4101:errorcluster)  [unwired: 4 in, 1 out]
                    n2446 = Bundle("MAIL SETTINGS"=w4096, "Auto Mail Send"=w4094, "TO (string):"=w4093) -> (w4095:T42)  [unwired: 1 in]
                    n2447 = Write to Binary File(file (use dialog)=w4102, data=w4095, error in=w4101) -> (refnum out=w4100:refnum<file>, error out=w4099:errorcluster)  [unwired: 3 in, 1 out]
                    n2448 = Close File(refnum=w4100, error in=w4099) -> (error out=w4098:errorcluster)  [unwired: 1 out]
                    n2449 = local write "data file error"(w4098) -> ()
                  }
                }
              }
            }
          }
          frame #17 {
            # "mail control"
            n2450 = local read "MAIL SETTINGS"() -> (w4119:T7)
            n2451 = local read "Auto Mail Send"() -> (w4105:bool)
            n2452 = Unbundle(w4119) -> ("OUT SERVER ADDRESS"=w4118:string, "FROM ACCOUNT"=w4117:string, "TEST MAIL"=w4116:bool)  [unwired: 4 out]
            n2453 = stacked-sequence {
              tunnel: "TO (string):" -> [_ w4158]
              tunnel: w4119 -> [w4124 w4157]
              tunnel: w4118 -> [w4123 w4156]
              tunnel: w4117 -> [w4122 w4155]
              tunnel: w4116 -> [w4121 _]
              tunnel: w4105 -> [_ w4154]
              tunnel: w4115 -> [_ w4153]
              tunnel: w4114 -> [_ w4152]
              tunnel: w4113 -> [_ w4151]
              tunnel: w4112 -> [_ w4150]
              tunnel: w4111 -> [_ w4149]
              tunnel: w4110 -> [_ w4148]
              tunnel: w4109 -> [_ w4147]
              tunnel: w4108 -> [_ w4146]
              tunnel: w4107 -> [_ w4145]
              tunnel: w4106 -> [_ w4144]
              tunnel: "TO (string):" -> [w4120 _]
              frame #0 {
                # "mail test"
                n2454 = case shown="True" w4121 {
                  tunnel: w4124 -> [_ w4128]
                  tunnel: w4120 -> [_ w4127]
                  tunnel: w4123 -> [_ w4126]
                  tunnel: w4122 -> [_ w4125]
                  frame False {
                  }
                  frame True {
                    n2455 = stacked-sequence {
                      seq-local: [_ _ w4138 _] -> [_ _ _ w4139]
                      tunnel: w4128 -> [w4131 _ _ w4143]
                      tunnel: w4127 -> [_ _ w4136 _]
                      tunnel: w4126 -> [_ _ w4134 _]
                      tunnel: w4125 -> [_ _ w4135 _]
                      frame #0 {
                        n2456 = Bundle(cluster=w4131, "TEST MAIL STATUS"="TEST START") -> (w4129:T7)  [unwired: 6 in]
                        n2457 = local write "MAIL SETTINGS"(w4129) -> ()
                      }
                      frame #1 {
                        n2458 = Wait (ms)(milliseconds to wait=500) -> ()  [unwired: 1 out]
                      }
                      frame #2 {
